vi "Stop.vi"(7 "Set? (f)":bool, 11 "In":bool) -> (3 "Out":bool)   [LabVIEW 2014, in "FgenPlugins.lvlib" / "DaqMx_Single.lvclass"]
uses:
  DaqMx_Single.lvclass
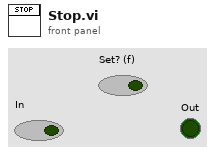
[diagram p1: front panel]
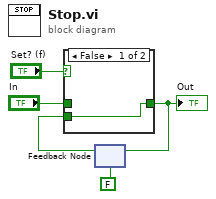
[diagram p0: block diagram]
diagram:
  n1 = feedback #1(FALSE ("In")) -> (w2:bool)
  n2 = case shown="False" "Set? (f)" {
    tunnel: "In" -> [_ w7]
    tunnel: [w6 w7] -> w3
    tunnel: w2 -> [w6 _]
    frame False {
    }
    frame True {
    }
  }
  "Out" <- w3
  n3 = feedback-in #1(w3) -> ()
